vi "Temp Sensor(IR)(SubVI).vi"(11 "tempIR_din":dbl) -> (1 "tempIR_out_range":bool, 2 "tempIR_max":dbl, 3 "tempIR":dbl, 4 "tempIR_min":dbl)   [LabVIEW 2017]
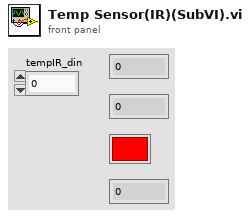
[diagram p1: front panel]
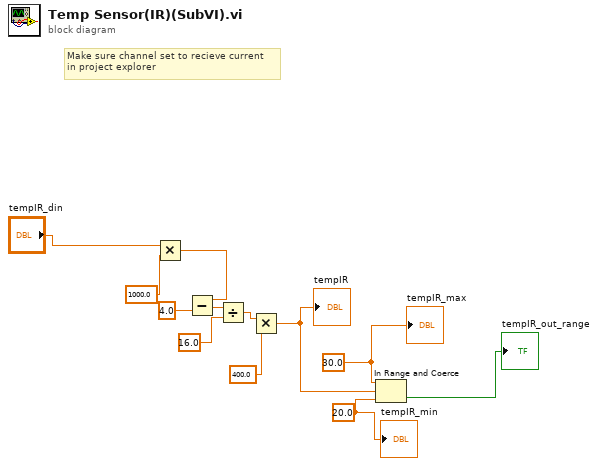
[diagram p0: block diagram]
diagram:
  w9 = 20.0
  w10 = 30.0
  # "Make sure channel set to recieve current\nin project explorer"
  n1 = Multiply(x="tempIR_din", y=1000.0) -> (x*y=w2:dbl)
  n2 = Subtract(x=w2, y=4.0) -> (x-y=w5:dbl)
  n3 = Divide(x=w5, y=16.0) -> (x/y=w7:dbl)
  n4 = Multiply(x=w7, y=400.0) -> (x*y=w12:dbl)
  "tempIR" <- w12
  n5 = In Range and Coerce(upper limit=w10, x=w12, lower limit=w9) -> (In Range?=→"tempIR_out_range":bool)  [unwired: 1 out]
  "tempIR_min" <- w9
  "tempIR_max" <- w10
